vi "WriteForceSubpanelDir.vi"(8 "error in (no error)":errorcluster, 10 "ForceSubpanelDir?":bool, 11 "SMO.UI.MAUI in":refnum<class "SMO.UI.MAUI.lvclass">) -> (0 "error out":errorcluster, 3 "SMO.UI.MAUI out":refnum<class "SMO.UI.MAUI.lvclass">)   [LabVIEW 2020, in "SMO.UI.MAUI.lvclass"]
uses:
  SMO.UI.MAUI.lvclass
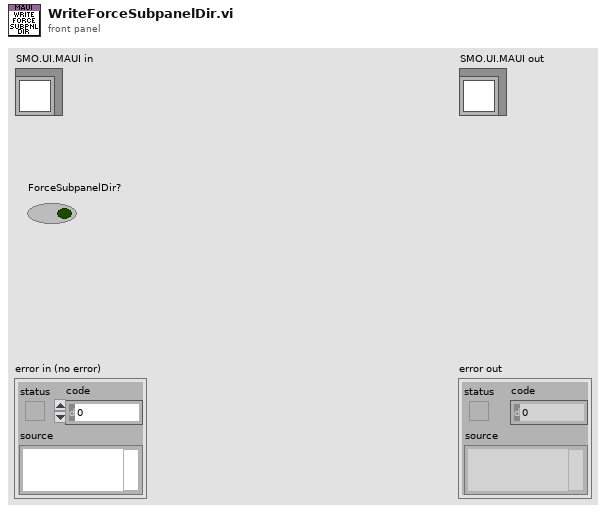
[diagram p1: front panel]
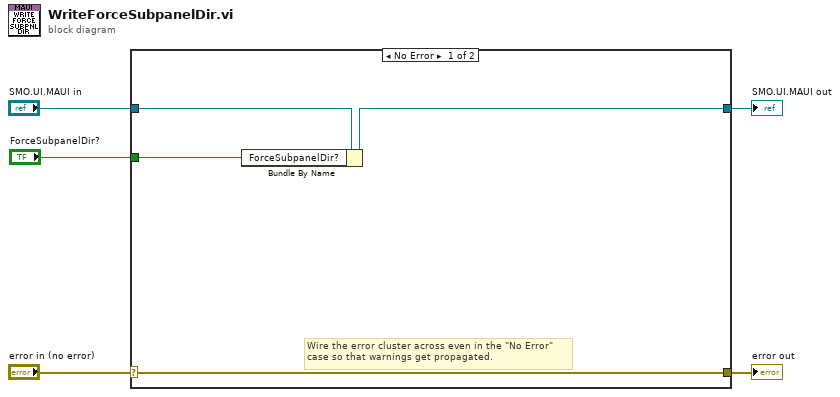
[diagram p0: block diagram]
diagram:
  n1 = case shown="No Error" "error in (no error)" {
    selector: "error in (no error)" -> [w9 w11]
    tunnel: [w9 w11] -> w4
    tunnel: [w8 w10] -> w2
    tunnel: "SMO.UI.MAUI in" -> [w7 w10]
    tunnel: "ForceSubpanelDir?" -> [w6 _]
    frame No Error {
      # "Wire the error cluster across even in the \"No Error\"\ncase so that warnings get propagated."
      n2 = Bundle By Name(cluster=w7, "ForceSubpanelDir?"=w6) -> (w8:refnum<class "SMO.UI.MAUI.lvclass">)
    }
    frame Error {
    }
  }
  "error out" <- w4
  "SMO.UI.MAUI out" <- w2
